vi "RDS Serial Handle Frame.vi"(8 "error in (no error)":errorcluster, 10 "RDS Serial Frame":refnum<class "RDS Serial Frame.lvclass">, 11 "RDS Serial Instrument Actor in":refnum<class "RDS Serial Instrument Actor.lvclass">) -> (0 "error out":errorcluster, 3 "RDS Serial Instrument Actor out":refnum<class "RDS Serial Instrument Actor.lvclass">)   [LabVIEW 2015, in "RDS Abstracts.lvlib" / "RDS Serial Instrument Actor.lvlib" / "RDS Serial Instrument Actor.lvclass"]
uses:
  RDS Serial Instrument Actor.lvclass
  Libraries/RDS Serial Handler/RDS Serial Frame.lvclass
  Libraries/RDS Child Messages/String Message/String Message.lvclass
  Libraries/RDS Framework/RDS Message ID.ctl
  Libraries/RDS Serial Handler/RDS Serial Frame.lvclass/RDS Serial Frame.ctl
  Libraries/RDS Child Messages/String Message/String Message.lvclass/String Message.ctl
  Libraries/RDS Framework/RDS Message Class/RDS Message.lvclass/RDS Message.ctl
  Libraries/RDS Framework/RDS Message Class/RDS Message.lvclass
  Libraries/RDS Child Messages/RDS Child Messages.lvlib
  RDS Parent Actor/RDS Parent Actor/RDS Parent Actor.lvclass
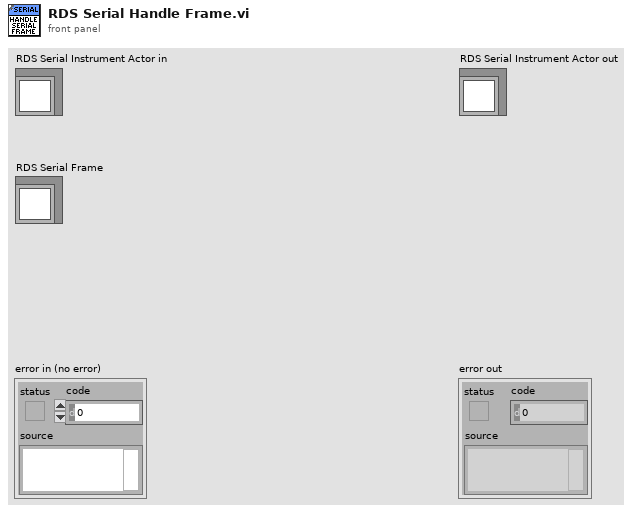
[diagram p1: front panel]
types:
  T1 = typedef "RDS Child Messages.lvlib/RDS Message ID.ctl" = enum16{"RDS Hello World", "String Message", "AIP_Status", "AIP_Command", "GPS_Data", "MCB_Command", "MCB_Status", "Compass_Data", "Depth_Data", "Battery_Data", "Contoller_State", "Set_Mag_Dev", "BTB_Shutdown", "State_Sample_Request", "State_Sample", "PID_Gains_Set", "Helm_Limiter_Set", "Helm_Heading_Command", "Helm_Steering_Command", "Helm_Status", "Controller_Message", "AIP_Set_Min_Depth", "Mission_Controller_State", "Mission_Upload", "Mission_Set_Op_and_Run", "Mission_Settings_Set"}
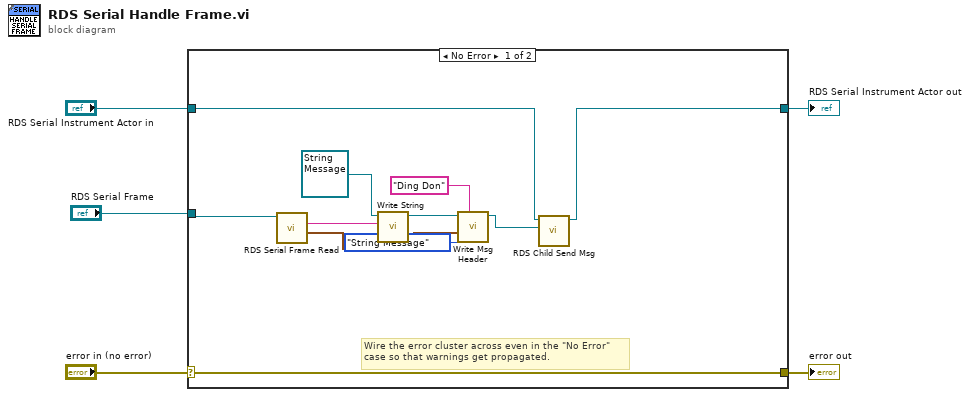
[diagram p0: block diagram]
diagram:
  n1 = case shown="No Error" "error in (no error)" {
    selector: "error in (no error)" -> [w16 w18]
    tunnel: [w16 w18] -> w4
    tunnel: [w6 w17] -> w2
    tunnel: "RDS Serial Instrument Actor in" -> [w7 w17]
    tunnel: "RDS Serial Frame" -> [w15 _]
    frame No Error {
      # "Wire the error cluster across even in the \"No Error\"\ncase so that warnings get propagated."
      n2 = call "RDS Serial Frame Read.vi"("RDS Serial Frame in"=w15) -> ("Time Stamp"=w11:timestamp, "Serial String"=w13:string)  [unwired: 7 in, 2 out]
      n3 = call "Write String.vi"("String"=w13, "String Message in"=refnum<class "String Message.lvclass"> refnum ("RDS Child Messages.lvlib:String Message.lvclass")) -> ("String Message out"=w12:refnum<class "String Message.lvclass">)  [unwired: 8 in, 1 out]
      n4 = call "Write Msg Header.vi"("Sender Name"="Ding Don", "Time Stamp"=w11, "Msg ID"=RDS_Message_ID."String Message", "RDS Message in"=w12) -> ("RDS Message out"=w8:refnum<class "String Message.lvclass">)  [unwired: 6 in, 1 out]
      n5 = call "RDS Child Send Msg.vi"("RDS Message"=w8, "RDS Parent Actor in"=w7) -> ("RDS Parent Actor out"=w6:refnum<class "RDS Serial Instrument Actor.lvclass">)  [unwired: 8 in, 1 out]
    }
    frame Error {
    }
  }
  "error out" <- w4
  "RDS Serial Instrument Actor out" <- w2
